vi "practicetest.vi"() -> ()   [LabVIEW 2018]
panel:
  out "Numeric 6":dbl
  out "Numeric 5":dbl
  out "Numeric 4":dbl
  out "Numeric 3":dbl
  out "Numeric 2":dbl
  out "Numeric":dbl
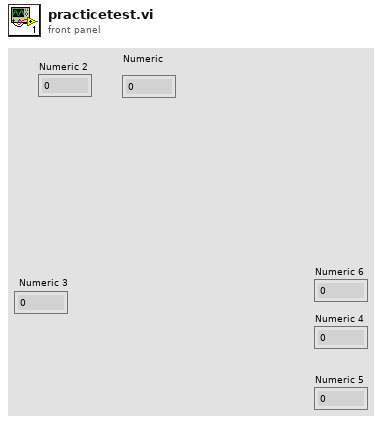
[diagram p1: front panel]
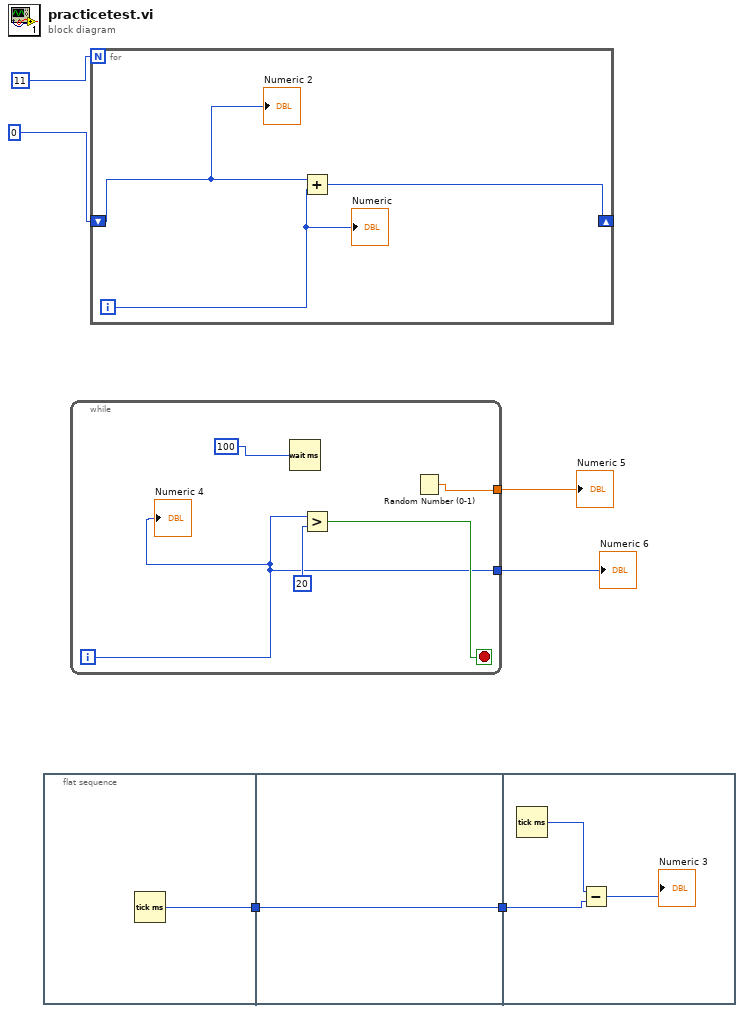
[diagram p0: block diagram]
diagram:
  n1 = flat-sequence {
    tunnel: [w7] -> w5
    tunnel: [w8] -> w6
    tunnel: w5 -> [w8]
    tunnel: w6 -> [w11]
    frame #0 {
      n2 = Tick Count (ms)() -> (millisecond timer value=w7:u32)
    }
    frame #1 {
    }
    frame #2 {
      n3 = Tick Count (ms)() -> (millisecond timer value=w10:u32)
      n4 = Subtract(x=w10, y=w11) -> (x-y=→"Numeric 3":u32)
    }
  }
  n5 = while {
    tunnel: [w14] -> w2
    tunnel: [w12] -> w1
    i -> [w12]
    stop <- w13 stop-if-true
    n6 = Wait (ms)(milliseconds to wait=100) -> ()  [unwired: 1 out]
    n7 = Greater?(x=w12, y=20) -> (0:w13:bool)
    n8 = Random Number (0-1)() -> (number: 0 to 1=w14:dbl)
    "Numeric 4" <- w12
  }
  "Numeric 5" <- w2
  "Numeric 6" <- w1
  n9 = for {
    N: 11 -> [_]
    shift-right: [w17] -> _
    shift-left: 0 -> [w18]
    i -> [w19]
    n10 = Add(x=w18, y=w19) -> (x+y=w17:i32)
    "Numeric" <- w19
    "Numeric 2" <- w18
  }
